vi "ESC_StdSci.vi"() -> ()   [LabVIEW 2015]
uses:
  SCI_DataPck.ctl
  SCI_DataType.ctl
  <vilib>/Instr/_visa.llb/VISA Configure Serial Port (Instr).vi
panel:
  in  "串口写数据包":T1={"包头"=170, "数据低8位"=0, "数据低高8位"=0, "数据类型"=0, "CRC余数"=0, "数据无效"=FALSE, "数据更新"=FALSE} {"包头" format="%02x"; "数据低8位" format="%02x"; "数据低高8位" format="%02x"; "数据类型" items=["SCIDP_SPTG1"=16, "SCIDP_SPTG2"=17, "SCIDP_INSTR1"=18, "SCIDP_INSTR2"=19, "SCIDP_DTTG1"=20, "SCIDP_DTTG2"=21, "SCIDP_VRPH1"=22, "SCIDP_VRPH2"=23, "RSVD0x18"=24, "RSVD0x19"=25, "RSVD0x1A"=26, "RSVD0x1B"=27, "RSVD0x1C"=28, "RSVD0x1D"=29, "RSVD0x1E"=30, "RSVD0x1F"=31, "SCIDP_SRVST1"=32, "SCIDP_SRVST2"=33, "SCIDP_SPFB1"=34, "SCIDP_SPFB2"=35, "RSVD0x24"=36, "RSVD0x25"=37, "RSVD0x26"=38, "RSVD0x27"=39, "RSVD0x28"=40, "RSVD0x29"=41, "RSVD0x2A"=42, "RSVD0x2B"=43, "RSVD0x2C"=44, "RSVD0x2D"=45, "SCIDP_EFFC1"=46, "SCIDP_EFFC2"=47, "RSVD0x30"=48, "RSVD0x31"=49, "SCIDP_IBUS1"=50, "SCIDP_IBUS2"=51, "SCIDP_IA1"=52, "SCIDP_IA2"=53, "SCIDP_IB1"=54, "SCIDP_IB2"=55, "SCIDP_IC1"=56, "SCIDP_IC2"=57, "SCIDP_UBUS1"=58, "SCIDP_UBUS2"=59, "SCIDP_TMPR1"=60, "SCIDP_TMPR2"=61, "RSVD0x3E"=62, "RSVD0x3F"=63, "VOID"=0]; "CRC余数" format="%02x"}
  in  "写入数据 2":u16 format="%x"
  in  "写入数据类型 2":u16 format="%x"
  in  "发送 2":bool
  out "写数据CRC余数 2":u16 format="%x"
  out "写数据更新":bool
  in  "停止按钮":bool
  in  "VISA资源名称":refnum<visa-resource-name>="COM1"
  out "串口更新":bool=TRUE
  out "串口读数据":i32[](array[numeric]) format="%04x"
  out "串口缓存空":bool
  out "串口缓存非空":bool
  out "串口写入数据 2":string
  in  "串口写入数据":string
  out "串口读数据包":T1={"包头"=170, "数据低8位"=0, "数据低高8位"=0, "数据类型"=0, "CRC余数"=0, "数据无效"=FALSE, "数据更新"=FALSE} {"包头" format="%02x"; "数据低8位" format="%02x"; "数据低高8位" format="%02x"; "数据类型" items=["SCIDP_SPTG1"=16, "SCIDP_SPTG2"=17, "SCIDP_INSTR1"=18, "SCIDP_INSTR2"=19, "SCIDP_DTTG1"=20, "SCIDP_DTTG2"=21, "SCIDP_VRPH1"=22, "SCIDP_VRPH2"=23, "RSVD0x18"=24, "RSVD0x19"=25, "RSVD0x1A"=26, "RSVD0x1B"=27, "RSVD0x1C"=28, "RSVD0x1D"=29, "RSVD0x1E"=30, "RSVD0x1F"=31, "SCIDP_SRVST1"=32, "SCIDP_SRVST2"=33, "SCIDP_SPFB1"=34, "SCIDP_SPFB2"=35, "RSVD0x24"=36, "RSVD0x25"=37, "RSVD0x26"=38, "RSVD0x27"=39, "RSVD0x28"=40, "RSVD0x29"=41, "RSVD0x2A"=42, "RSVD0x2B"=43, "RSVD0x2C"=44, "RSVD0x2D"=45, "SCIDP_EFFC1"=46, "SCIDP_EFFC2"=47, "RSVD0x30"=48, "RSVD0x31"=49, "SCIDP_IBUS1"=50, "SCIDP_IBUS2"=51, "SCIDP_IA1"=52, "SCIDP_IA2"=53, "SCIDP_IB1"=54, "SCIDP_IB2"=55, "SCIDP_IC1"=56, "SCIDP_IC2"=57, "SCIDP_UBUS1"=58, "SCIDP_UBUS2"=59, "SCIDP_TMPR1"=60, "SCIDP_TMPR2"=61, "RSVD0x3E"=62, "RSVD0x3F"=63, "VOID"=0]; "CRC余数" format="%02x"}
  in  "读出数据类型":u16=16 format="%02x"
  out "读数据CRC余数":u16 format="%x"
  out "读出数据":u16 format="%x"
  out "包头":u16 format="%x"
  out "串口预写入数据":string
  out "串口预写入簇":T1={"包头"=170, "数据低8位"=0, "数据低高8位"=0, "数据类型"=0, "CRC余数"=0, "数据无效"=FALSE, "数据更新"=FALSE} {"包头" format="%02x"; "数据低8位" format="%02x"; "数据低高8位" format="%02x"; "数据类型" items=["SCIDP_SPTG1"=16, "SCIDP_SPTG2"=17, "SCIDP_INSTR1"=18, "SCIDP_INSTR2"=19, "SCIDP_DTTG1"=20, "SCIDP_DTTG2"=21, "SCIDP_VRPH1"=22, "SCIDP_VRPH2"=23, "RSVD0x18"=24, "RSVD0x19"=25, "RSVD0x1A"=26, "RSVD0x1B"=27, "RSVD0x1C"=28, "RSVD0x1D"=29, "RSVD0x1E"=30, "RSVD0x1F"=31, "SCIDP_SRVST1"=32, "SCIDP_SRVST2"=33, "SCIDP_SPFB1"=34, "SCIDP_SPFB2"=35, "RSVD0x24"=36, "RSVD0x25"=37, "RSVD0x26"=38, "RSVD0x27"=39, "RSVD0x28"=40, "RSVD0x29"=41, "RSVD0x2A"=42, "RSVD0x2B"=43, "RSVD0x2C"=44, "RSVD0x2D"=45, "SCIDP_EFFC1"=46, "SCIDP_EFFC2"=47, "RSVD0x30"=48, "RSVD0x31"=49, "SCIDP_IBUS1"=50, "SCIDP_IBUS2"=51, "SCIDP_IA1"=52, "SCIDP_IA2"=53, "SCIDP_IB1"=54, "SCIDP_IB2"=55, "SCIDP_IC1"=56, "SCIDP_IC2"=57, "SCIDP_UBUS1"=58, "SCIDP_UBUS2"=59, "SCIDP_TMPR1"=60, "SCIDP_TMPR2"=61, "RSVD0x3E"=62, "RSVD0x3F"=63, "VOID"=0]; "CRC余数" format="%02x"}
  in  "数据包 1st":T1={"包头"=170, "数据低8位"=0, "数据低高8位"=0, "数据类型"=0, "CRC余数"=0, "数据无效"=FALSE, "数据更新"=FALSE} {"包头" format="%02x"; "数据低8位" format="%02x"; "数据低高8位" format="%02x"; "数据类型" items=["SCIDP_SPTG1"=16, "SCIDP_SPTG2"=17, "SCIDP_INSTR1"=18, "SCIDP_INSTR2"=19, "SCIDP_DTTG1"=20, "SCIDP_DTTG2"=21, "SCIDP_VRPH1"=22, "SCIDP_VRPH2"=23, "RSVD0x18"=24, "RSVD0x19"=25, "RSVD0x1A"=26, "RSVD0x1B"=27, "RSVD0x1C"=28, "RSVD0x1D"=29, "RSVD0x1E"=30, "RSVD0x1F"=31, "SCIDP_SRVST1"=32, "SCIDP_SRVST2"=33, "SCIDP_SPFB1"=34, "SCIDP_SPFB2"=35, "RSVD0x24"=36, "RSVD0x25"=37, "RSVD0x26"=38, "RSVD0x27"=39, "RSVD0x28"=40, "RSVD0x29"=41, "RSVD0x2A"=42, "RSVD0x2B"=43, "RSVD0x2C"=44, "RSVD0x2D"=45, "SCIDP_EFFC1"=46, "SCIDP_EFFC2"=47, "RSVD0x30"=48, "RSVD0x31"=49, "SCIDP_IBUS1"=50, "SCIDP_IBUS2"=51, "SCIDP_IA1"=52, "SCIDP_IA2"=53, "SCIDP_IB1"=54, "SCIDP_IB2"=55, "SCIDP_IC1"=56, "SCIDP_IC2"=57, "SCIDP_UBUS1"=58, "SCIDP_UBUS2"=59, "SCIDP_TMPR1"=60, "SCIDP_TMPR2"=61, "RSVD0x3E"=62, "RSVD0x3F"=63, "VOID"=0]; "CRC余数" format="%02x"}
  in  "写入数据":u16 format="%x"
  in  "写入数据类型":u16 format="%x"
  in  "发送":bool
  out "写数据CRC余数":u16 format="%x"
  out "串口读缓存字符数":u32
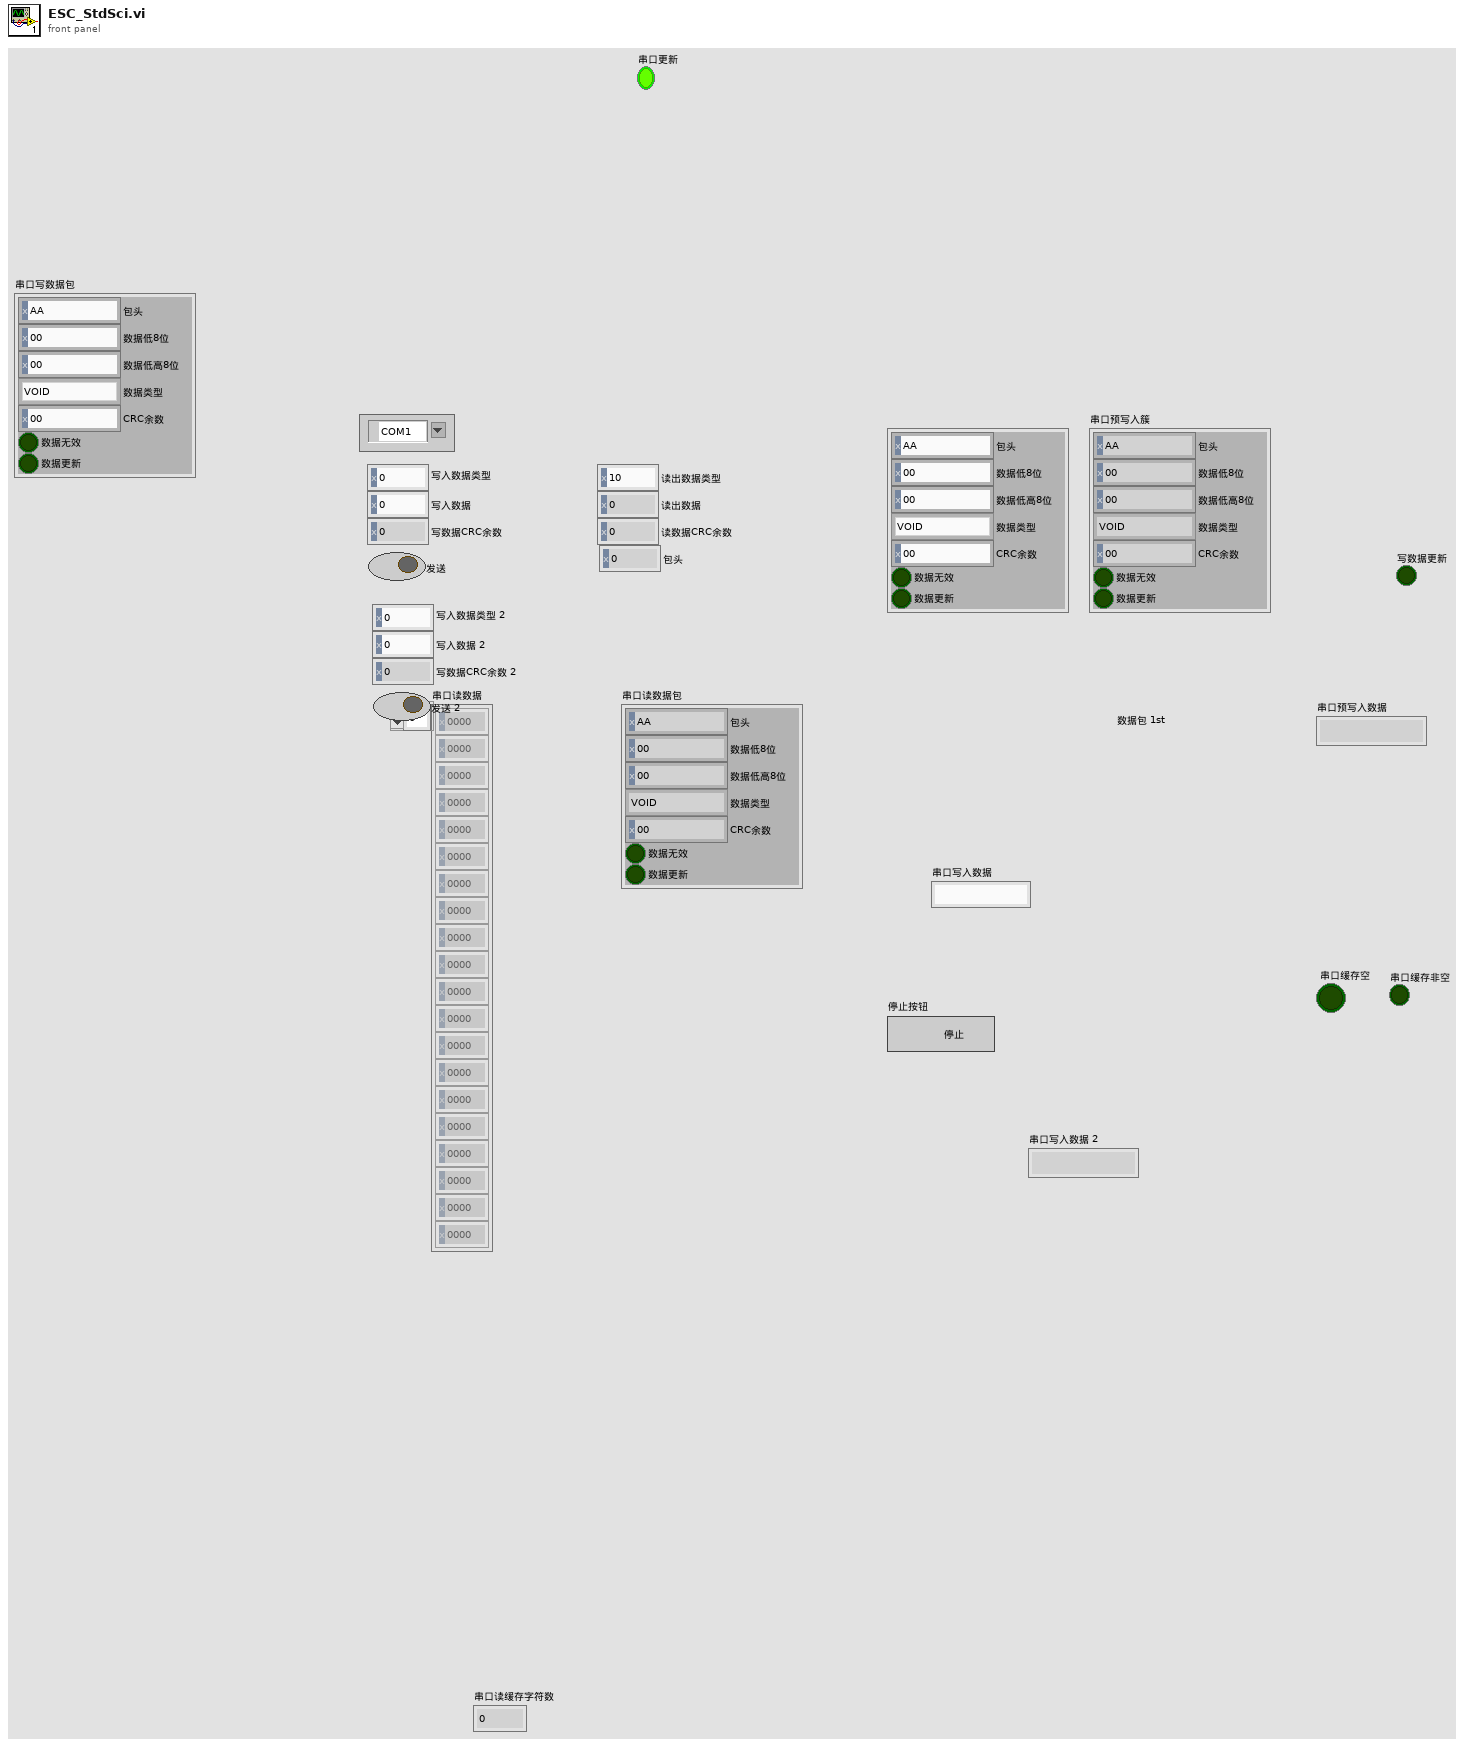
[diagram p1: front panel]
types:
  T1 = typedef "SCI_DataPck.ctl" = cluster{"包头":u16, "数据低8位":u16, "数据低高8位":u16, "数据类型":T2, "CRC余数":u16, "数据无效":bool, "数据更新":bool}
  T2 = typedef "SCI_DataType.ctl" = u16
  T3 = cluster{"波特率":u32, "数据比特":u16, "奇偶":enum16{"None", "Odd", "Even", "Mark", "Space"}, "停止位":u16, "流控制":u16}
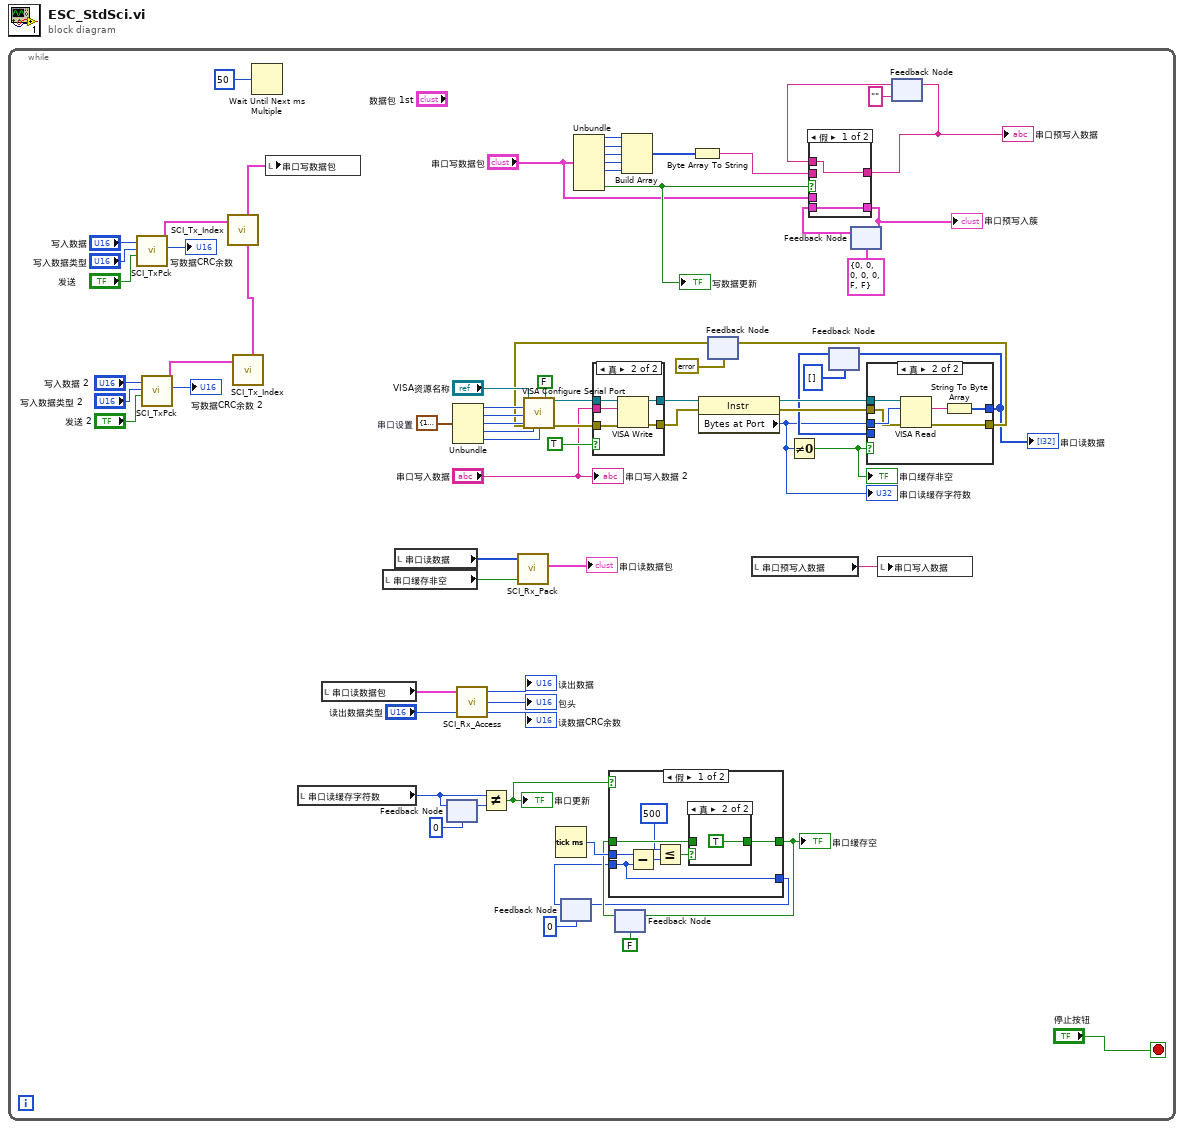
[diagram p0: block diagram]
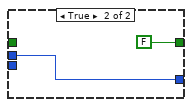
[diagram p5: hidden frame]
diagram:
  n1 = while {
    stop <- "停止按钮" stop-if-true
    w65 = T3 {"波特率"=115200, "数据比特"=8, "奇偶"=enum."None", "停止位"=10, "流控制"=0}  # 串口设置
    n2 = call "SCI_TxPck.vi"("数据有效"="发送", "数据类型"="写入数据类型", "数据"="写入数据") -> ("CRC余数"=→"写数据CRC余数":u16, "数据包输出"=w14:T1)  [unwired: 7 in]
    n3 = call "SCI_TxPck.vi"("数据有效"="发送 2", "数据类型"="写入数据类型 2", "数据"="写入数据 2") -> ("CRC余数"=→"写数据CRC余数 2":u16, "数据包输出"=w8:T1)  [unwired: 7 in]
    n4 = call "SCI_Tx_Index.vi"("输入数据包（簇）"=w8) -> ("上一个包数据（簇）"=w3:T1)  [unwired: 10 in]
    n5 = call "SCI_Tx_Index.vi"("下一包数据（簇）"=w3, "输入数据包（簇）"=w14) -> ("上一个包数据（簇）"=w1:T1)  [unwired: 9 in]
    n6 = Wait Until Next ms Multiple(millisecond multiple=50) -> ()  [unwired: 1 out]
    n7 = local write "串口写数据包"(w1) -> ()
    n8 = local read "串口读缓存字符数"() -> (w20:u32)
    n9 = local read "串口读数据包"() -> (w50:T1)
    n10 = local read "串口缓存非空"() -> (w53:bool)
    n11 = local read "串口读数据"() -> (w54:i32[])
    n12 = feedback #1(u32 0 ("Bytes at Port")) -> (w31:u32)
    n13 = feedback-in #1(w20) -> ()
    n14 = Unbundle(w65) -> ("波特率"=w70:u32, "数据比特"=w69:u16, "奇偶"=w68:enum16{"None", "Odd", "Even", "Mark", "Space"}, "停止位"=w67:u16, "流控制"=w66:u16)
    n15 = call "SCI_Rx_Access.vi"("数据类型"="读出数据类型", "串口读数据包（簇）"=w50) -> ("CRC余数"=→"读数据CRC余数":u16, "包头"=→"包头":u16, "数据输出"=→"读出数据":u16)  [unwired: 1 in]
    n16 = Not Equal?(x=w20, y=w31) -> (x != y?=w56:bool)
    "串口更新" <- w56
    n17 = call "SCI_Rx_Pack.vi"("确认"=w53, "SCI RX数据块"=w54) -> ("SciPckOut"=→"串口读数据包":T1)  [unwired: 5 in, 1 out]
    n18 = Tick Count (ms)() -> (millisecond timer value=w57:u32)
    n19 = feedback #2(u32 0 ("Bytes at Port")) -> (w21:u32)
    n20 = Unbundle("串口写数据包") -> ("包头"=w45:u16, "数据低8位"=w44:u16, "数据低高8位"=w43:u16, "数据类型"=w42:T2, "CRC余数"=w41:u16, "数据更新"=w32:bool)  [unwired: 1 out]
    "写数据更新" <- w32
    n21 = feedback #3(FALSE) -> (w24:bool)
    n22 = case shown="假" w56 {
      tunnel: [w89 w95] -> w22
      tunnel: w57 -> [w91 w95]
      tunnel: w21 -> [w89 _]
      tunnel: [w87 FALSE ("crossing")] -> w25
      tunnel: w24 -> [w88 _]
      frame False {
        n23 = Subtract(x=w91, y=w89) -> (x-y=w86:u32)
        n24 = Less Or Equal?(x=500, y=w86) -> (x <= y?=w90:bool)
        n25 = case shown="真" w90 {
          tunnel: w88 -> [w92 _]
          tunnel: [w92 TRUE ("crossing")] -> w87
          frame False {
          }
          frame True {
          }
        }
      }
      frame True {
      }
    }
    "串口缓存空" <- w25
    n26 = feedback-in #2(w22) -> ()
    n27 = feedback-in #3(w25) -> ()
    n28 = Build Array(w45, w44, w43, w42, w41) -> (w40:T2[])
    n29 = Byte Array To String(unsigned byte array=w40) -> (string=w12:string)
    n30 = feedback #4(errorcluster {"status"=FALSE, "code"=0, "source"=""} ("error out")) -> (w33:errorcluster)
    n31 = call-poly "VISA Configure Serial Port"("VISA resource name"="VISA资源名称", "Enable Termination\nChar (T)"=FALSE, "baud rate (9600)"=w70, "data bits (8)"=w69, "parity (0:none)"=w68, "error in (no error)"=w33, "stop bits (10: 1 bit)"=w67, "flow control (0:none)"=w66) -> ("VISA resource name out"=w61:refnum<visa-resource-name>, "error out"=w64:errorcluster)  [unwired: 1 in, 5 out]
    n32 = case shown="真" TRUE {
      tunnel: w64 -> [w74 w80]
      tunnel: [w74 w79] -> w63
      tunnel: [w75 w78] -> w62
      tunnel: w61 -> [w75 w77]
      tunnel: "串口写入数据" -> [_ w76]
      frame False {
      }
      frame True {
        n33 = VISA Write(VISA resource name=w77, write buffer=w76, error in (no error)=w80) -> (VISA resource name out=w78:refnum<visa-resource-name>, error out=w79:errorcluster)  [unwired: 1 out]
      }
    }
    n34 = property class="Instr"(reference=w62, error in=w63) -> (reference out=w60:refnum<visa-resource-name>, error out=w59:errorcluster, "Bytes at Port"=w19:u32)
    "串口读缓存字符数" <- w19
    n35 = local read "串口预写入数据"() -> (w9:string)
    n36 = Not Equal To 0?(x=w19) -> (x != 0?=w58:bool)
    "串口缓存非空" <- w58
    n37 = feedback #5(u8[] [] ("unsigned byte array")) -> (w27:u8[])
    n38 = feedback #6(T1 {"包头"=0, "数据低8位"=0, "数据低高8位"=0, "数据类型"=0, "CRC余数"=0, "数据无效"=FALSE, "数据更新"=FALSE}) -> (w37:T1)
    n39 = case shown="真" w58 {
      tunnel: w27 -> [w97 _]
      tunnel: [w97 w100] -> w28
      tunnel: w60 -> [_ w102]
      tunnel: w19 -> [_ w101]
      tunnel: w59 -> [w96 w99]
      tunnel: [w96 w98] -> w52
      frame False {
      }
      frame True {
        n40 = VISA Read(VISA resource name=w102, byte count=w101, error in (no error)=w99) -> (read buffer=w103:string, error out=w98:errorcluster)  [unwired: 2 out]
        n41 = String To Byte Array(string=w103) -> (unsigned byte array=w100:u8[])
      }
    }
    "串口读数据" <- w28
    n42 = feedback-in #4(w52) -> ()
    n43 = feedback-in #5(w28) -> ()
    n44 = local write "串口写入数据"(w9) -> ()
    n45 = feedback #7("" ("string")) -> (w13:string)
    n46 = case shown="假" w32 {
      tunnel: "串口写数据包" -> [_ w84]
      tunnel: [w82 w84] -> w38
      tunnel: w37 -> [w82 _]
      tunnel: w13 -> [w81 _]
      tunnel: [w81 w83] -> w11
      tunnel: w12 -> [_ w83]
      frame False {
      }
      frame True {
      }
    }
    "串口预写入数据" <- w11
    "串口预写入簇" <- w38
    n47 = feedback-in #6(w38) -> ()
    n48 = feedback-in #7(w11) -> ()
    "串口写入数据 2" <- "串口写入数据"
  }
